vi "Convert LV-DB Types.vi"(7 "conversion":enum16{"LV to DB", "DB to LV"}(ring), 8 "error in":errorcluster, 10 "DataType":string="I64") -> (0 "error out":errorcluster, 2 "Converted Type":string="I64")   [LabVIEW 2018, in "Serializer.lvclass"]
uses:
  Serializer.lvclass
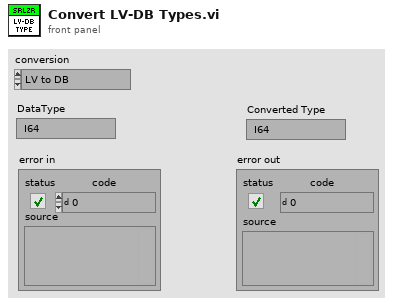
[diagram p1: front panel]
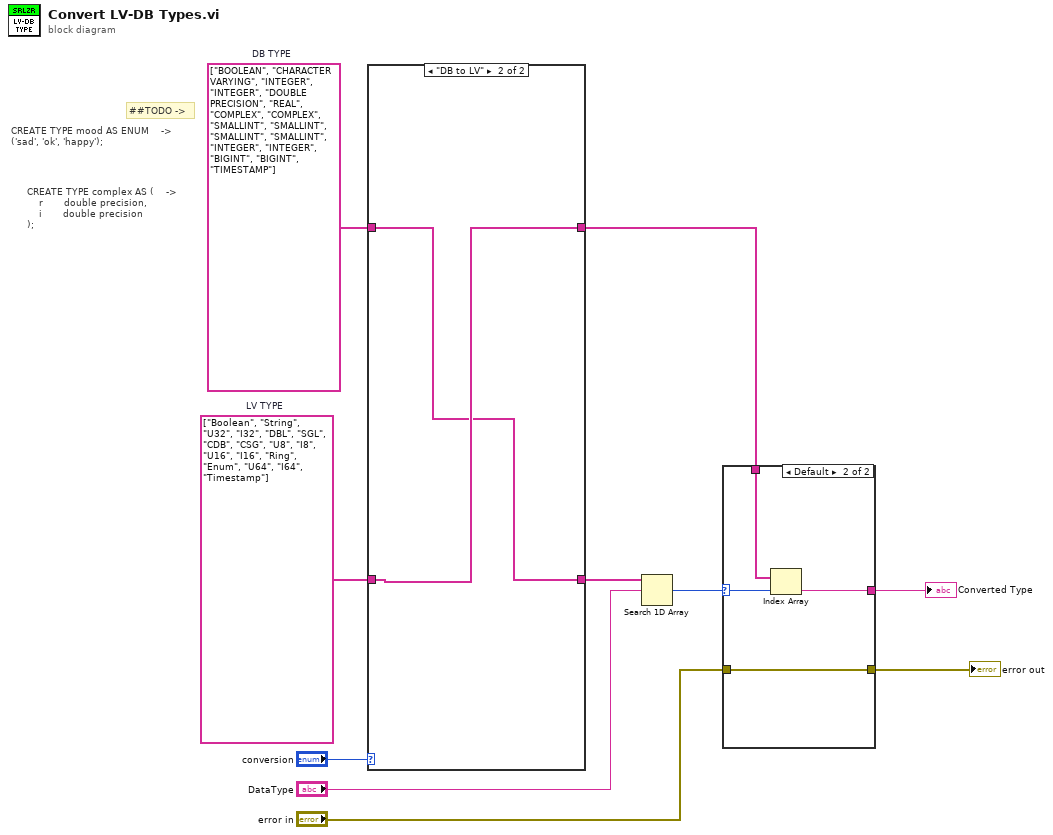
[diagram p0: block diagram]
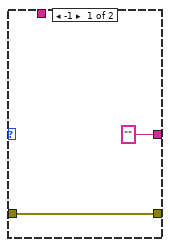
[diagram p2: hidden frame]
diagram:
  w5 = string[] ["BOOLEAN", "CHARACTER VARYING", "INTEGER", "INTEGER", "DOUBLE PRECISION", "REAL", "COMPLEX", "COMPLEX", "SMALLINT", "SMALLINT", "SMALLINT", "SMALLINT", "INTEGER", "INTEGER", "BIGINT", "BIGINT", "TIMESTAMP"]  # DB TYPE
  w6 = string[] ["Boolean", "String", "U32", "I32", "DBL", "SGL", "CDB", "CSG", "U8", "I8", "U16", "I16", "Ring", "Enum", "U64", "I64", "Timestamp"]  # LV TYPE
  # "CREATE TYPE mood AS ENUM    ->\n('sad', 'ok', 'happy');"
  # "CREATE TYPE complex AS (    ->\n    r       double precision,\n    i       double precision\n);"
  # "##TODO ->"
  n1 = case shown="\"DB to LV\"" "conversion" {
    tunnel: [w12 w13] -> w9
    tunnel: w6 -> [w12 w14]
    tunnel: w5 -> [w11 w13]
    tunnel: [w11 w14] -> w4
    frame "LV to DB" {
    }
    frame "DB to LV" {
    }
  }
  n2 = Search 1D Array(1D array=w9, element="DataType") -> (index of element=w7:i32)  [unwired: 1 in]
  n3 = case shown="Default" w7 {
    selector: w7 -> [_ w19]
    tunnel: w4 -> [_ w20]
    tunnel: ["" w18] -> w3
    tunnel: [w15 w17] -> w2
    tunnel: "error in" -> [w15 w17]
    frame -1 {
    }
    frame Default {
      n4 = Index Array(array=w20, index=w19) -> (element=w18:string)
    }
  }
  "Converted Type" <- w3
  "error out" <- w2
